vi "SubPanel_Remove.vi"(8 "Error":errorcluster, 11 "SubPanel":refnum<vi>) -> (0 "Error Out":errorcluster, 2 "Removed":bool, 3 "SubPanel Out":refnum<vi>)   [LabVIEW 2020]
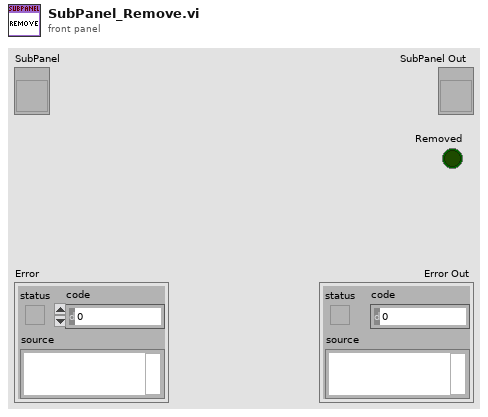
[diagram p1: front panel]
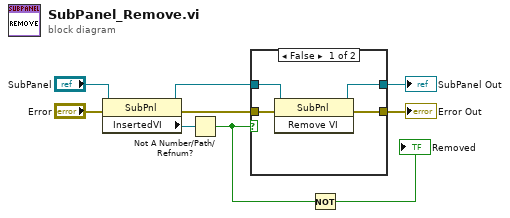
[diagram p0: block diagram]
diagram:
  n1 = property class="SubPnl"(reference="SubPanel", error in="Error") -> (reference out=w6:refnum<vi>, error out=w4:errorcluster, "InsertedVI"=w3:refnum<vi>)
  n2 = Not A Number/Path/Refnum?(number/path/refnum=w3) -> (NaN/Path/Refnum?=w2:bool)
  n3 = case shown="False" w2 {
    tunnel: [w13 w15] -> w9
    tunnel: [w12 w14] -> w8
    tunnel: w6 -> [w11 w14]
    tunnel: w4 -> [w10 w15]
    frame False {
      n4 = invoke class="SubPnl" method="Remove VI"(reference=w11, error in=w10) -> (reference out=w12:refnum<vi>, error out=w13:errorcluster)  [unwired: 1 in, 1 out]
    }
    frame True {
    }
  }
  "Error Out" <- w9
  "SubPanel Out" <- w8
  n5 = Not(x=w2) -> (.not. x?=→"Removed":bool)
